vi "STAGE+mono+counter_edit21.vi"() -> ()   [LabVIEW 2017]
panel:
  out "Timeout":bool
  out "PROGRESS":u8(slide) max=10 step=10 scale=0.0..1.0
  in  "?":enum32{"Scan Data", "Scans", "RT Data"}(tab)
  out "XY Graph":cluster{dbl[], dbl[]}(graph)
  out "XY Graph 2":cluster{dbl[], dbl[]}[](graph)
  in  "Collect Data!":bool
  out "Waveform Graph":waveform(dbl)[](graph)
  out "?":i32(knob) scale=0.0..1000000.0
  out "Photon Counts":dbl
  in  "Wavelength":dbl
  in  "Show Real Time Data":bool
  in  "?":enum32{"DELAY", "COUNTER", "MONO", "PLOT"}(tab)
  out "Final time [ps]":dbl
  out "Current time [ps]":dbl
  out "Initial time [ps]":dbl
  in  "Set this as t0":bool
  in  "Axis":i32=1
  in  "Motor ON":bool
  in  "Motor OFF":bool
  out "Current Position [mm]":dbl
  out "Final Position [mm]":dbl
  in  "Data Points":i32=100
  out "Current Point":i32
  in  "Step Size [um]":i32=10
  in  "Target [mm]":dbl format="%.3f"
  in  "Move":bool
  out "Initial position [mm]":dbl
  in  "GPIB address":string="23"
  in  "Count Mode":u16(ring) items=["A,B for Preset T", "A-B for Preset T", "A+B for Preset T", "A for Preset B"]
  in  "Trigger mode":u16(ring) items=["10 MHz"=0, "Input 2"=2, "Input T"=3]
  in  "Channel A Input":u16(ring)=1 items=["10 MHz", "Input 1"]
  in  "Channel B Input":u16(ring)=2 items=["Input 1"=1, "Input 2"=2]
  in  "Number of Measurements\n to take at one point/ Number of Periods":u16=1 min=1 max=2000 step=1
  in  "Time between measurements\n at one point (s)/Dwell Time":dbl=0.002 min=0.002 max=60.0 step=0.001
  in  "gate mode (CW:0)":i16(slide) scale=0.0..2.0 scale format="%.2f"
  out "Counts":i32
  in  "Integrating time \nin 10^-7 sec":dbl=10000000.0
  in  "Discriminator Level (mV)":dbl min=-300.0 max=300.0 step=0.2
  in  "Discriminator Slope":bool
  in  "Channel":i16 min=0 max=2 step=1
  out "Grating #":dbl
  out "Blaze angle":dbl
  out "Grooves/mm":dbl
  out "Mono port":T1(ring)
  out "Time delay":u32=450000 min=1
  in  "Step size":dbl=10.0 min=0.0
  in  "Scan to":i32=4000
  in  "Scan from":i32=2600
  out "Current wavelength":dbl
  in  "?":bool
  in  "Array":dbl[](array[numeric])
  out "Numeric":i32
  out "Numeric 2":i32
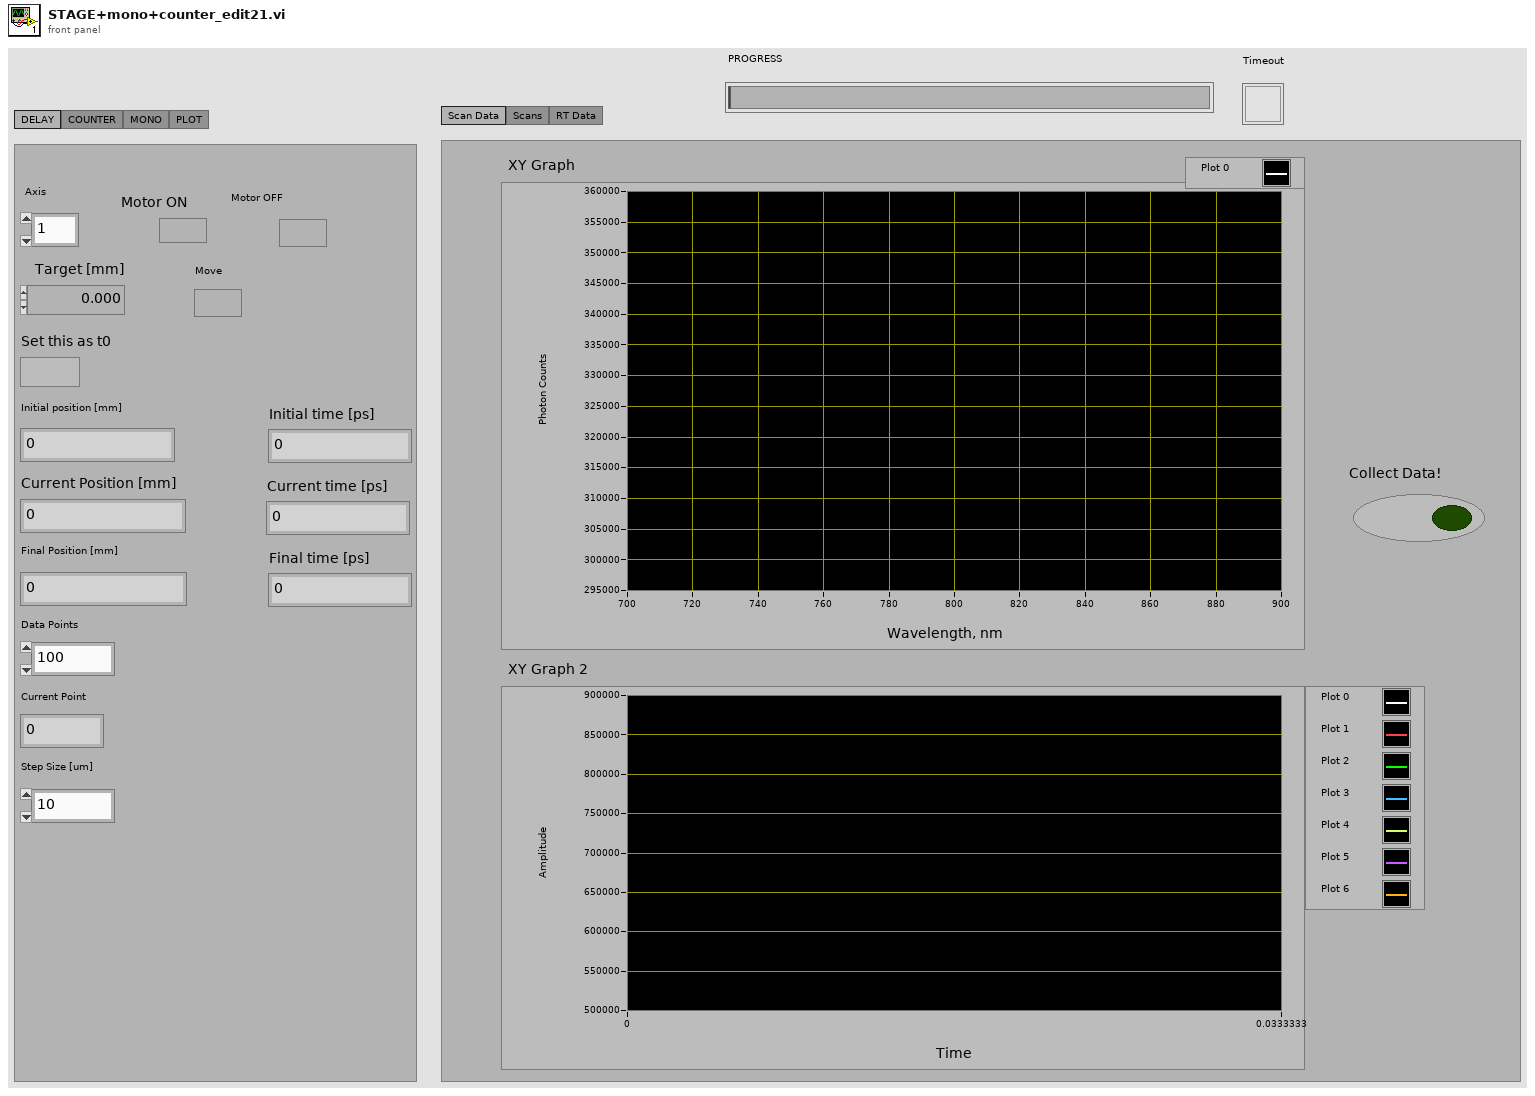
[diagram p1: front panel]
types:
  T1 = enum8{"COM 1", "COM 2", "COM 3", "COM 4", "COM 5", "COM 6", "COM 7", "COM 8", "COM 9"}
  T2 = cluster{"input XON/XOFF":bool, "input HW Handshake":bool, "input alt HW HShk":bool, "output XON/XOFF":bool, "output HW Handshake":bool, "output alt HW HShk":bool, "XOFF byte":u8, "XON byte":u8, "parity error byte":u16}
  T3 = enum16{"no parity", "odd parity", "even parity", "mark parity", "space parity"}
  T4 = typedef "NI_Matrix.lvlib/RealMatrix.ctl" = dbl[][]
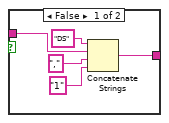
[diagram p3: hidden frame]
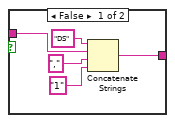
[diagram p5: hidden frame]
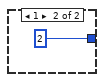
[diagram p9: hidden frame]
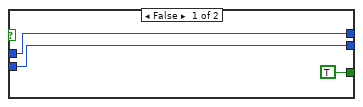
[diagram p10: hidden frame]
diagram:
  (unwired) FALSE
  w28 = u32 19200  # baud rate
  w27 = u16 8  # data bits
  w26 = enum16{"1 bit", "1.5 bits", "2 bits"}."1 bit"  # stop bits
  w30 = T3."no parity"  # parity
  w6 = 4  # 0=COM1 so n=COM(n+1)
  w29 = u16 1024  # buffer size
  n1 = flat-sequence {
    tunnel: [w33] -> w21
    tunnel: [w32] -> w20
    frame #0 {
      n2 = call "CM Com Read ini.vi"() -> ("Mono port"=w32:T1, "time delay1"=w33:u32)  [unwired: 7 in]
    }
  }
  n3 = call "CM Serial Port Setup.vi"("COM port"=w20, "time delay"=w21) -> ("time delay1"=w16:u32, "DK port Out"=w17:T1, "error code"=w19:i32)  [unwired: 7 in]
  n4 = Equal To 0?(x=w19) -> (x = 0?=w18:bool)
  n5 = case shown="True" w18 {
    tunnel: w17 -> [w36 w39]
    tunnel: w16 -> [w35 w38]
    tunnel: [w36 w39] -> w3
    tunnel: [w35 w38] -> w2
    tunnel: [TRUE FALSE] -> w1
    frame False {
    }
    frame True {
      n6 = call "CM Com Write ini.vi"("time delay1"=w39, "Mono port"=w38) -> ()  [unwired: 7 in]
      n7 = local write "Mono port"(w39) -> ()
      n8 = local write "Time delay"(w38) -> ()
    }
  }
  n9 = call <vilib>:"Serial Port Init.vi"("flow control etc."=T2 {"input XON/XOFF"=FALSE, "input HW Handshake"=FALSE, "input alt HW HShk"=FALSE, "output XON/XOFF"=FALSE, "output HW Handshake"=FALSE, "output alt HW HShk"=FALSE, "XOFF byte"=13, "XON byte"=11, "parity error byte"=0}, "parity"=w30, "buffer size"=w29, "stop bits"=w26, "data bits"=w27, "baud rate"=w28, "port number"=w6) -> ("error code"=w25:i32)
  n10 = Concatenate Strings("\r", "\n") -> (w22:string)
  n11 = while {
    tunnel: w2 -> [w42]
    tunnel: w3 -> [w41]
    stop <- TRUE continue-if-true
    n12 = case shown="True" "?" {
      tunnel: w42 -> [_ w45]
      tunnel: w41 -> [_ w44]
      frame False {
      }
      frame True {
        n13 = Two Button Dialog(message="Do you want to change grating?", 1:"No" ("F button name (\"Cancel\")"), 2:"Yes" ("T button name (\"OK\")")) -> (T button?=w46:bool)
        n14 = case shown="True" w46 {
          tunnel: w45 -> [_ w51]
          tunnel: w44 -> [_ w50]
          frame False {
          }
          frame True {
            n15 = Two Button Dialog(message="Disable voltage from PMT", 1:"Do not swich grating" ("F button name (\"Cancel\")"), 2:"Done" ("T button name (\"OK\")")) -> (T button?=w52:bool)
            n16 = case shown="True" w52 {
              tunnel: w51 -> [_ w64]
              tunnel: w50 -> [_ w63]
              frame False {
              }
              frame True {
                n17 = flat-sequence {
                  tunnel: w64 -> [w68]
                  tunnel: [w68] -> w58
                  tunnel: w63 -> [w67]
                  tunnel: [w67] -> w57
                  tunnel: [w65] -> w56
                  tunnel: w58 -> [w73]
                  tunnel: [w73] -> w61
                  tunnel: w57 -> [w74]
                  tunnel: [w74] -> w60
                  tunnel: w56 -> [w72]
                  tunnel: [w72] -> w59
                  tunnel: w61 -> [w78]
                  tunnel: w60 -> [w79]
                  tunnel: [w77] -> w62
                  tunnel: w59 -> [w77]
                  frame #0 {
                    n18 = local read "Grating #"() -> (w66:dbl)
                    n19 = case shown="2, Default" w66 {
                      tunnel: [1 2] -> w65
                      frame 2, Default {
                      }
                      frame 1 {
                      }
                    }
                    n20 = call "Select11x2.vi"("time delay"=w68, "NEW GRT?"=w65, "port number"=w67) -> ()  [unwired: 3 out]
                  }
                  frame #1 {
                    n21 = call "Query11x.vi"("port number"=w74, "QUERY"=u16 2, "time delay"=w73) -> ("STATUS MESSAGE"=w71:u16)  [unwired: 3 out]
                    n22 = local write "Grooves/mm"(w71) -> ()
                  }
                  frame #2 {
                    n23 = Divide(x=w78, y=i16 100 ("device (1)")) -> (x/y=w80:dbl)
                    n24 = call "Query11x.vi"("port number"=w79, "QUERY"=u16 3, "time delay"=w80) -> ("STATUS MESSAGE"=w76:u16)  [unwired: 3 out]
                    n25 = local write "Blaze angle"(w76) -> ()
                  }
                }
                n26 = local write "Grating #"(w62) -> ()
              }
            }
          }
        }
      }
    }
  }
  n27 = while {
    tunnel: w6 -> [w97]
    tunnel: w22 -> [w98]
    tunnel: w25 -> [_]
    tunnel: "Axis" -> [w95]
    stop <- TRUE continue-if-true
    w96 = u32 200  # timeout
    n28 = Format Into String(w95) -> (resulting string=w99:string)  [unwired: 3 in, 1 out]
    n29 = flat-sequence {
      tunnel: w99 -> [w104]
      tunnel: w98 -> [w103]
      tunnel: w97 -> [w105]
      tunnel: w96 -> [w102]
      tunnel: [w104] -> w94
      tunnel: [w103] -> w93
      tunnel: [w105] -> w92
      tunnel: [w102] -> w91
      tunnel: w94 -> [w115]
      tunnel: w93 -> [w114]
      tunnel: w92 -> [w116]
      tunnel: w91 -> [w112]
      tunnel: [w115] -> w90
      tunnel: [w114] -> w89
      tunnel: [w116] -> w88
      tunnel: [w112] -> w87
      tunnel: w90 -> [w125]
      tunnel: w89 -> [w124]
      tunnel: w88 -> [w126]
      tunnel: w87 -> [w122]
      tunnel: [w125] -> w86
      tunnel: [w124] -> w85
      tunnel: [w126] -> w84
      tunnel: [w122] -> w83
      tunnel: w86 -> [w138]
      tunnel: w85 -> [w135]
      tunnel: w84 -> [w137]
      tunnel: w83 -> [w136]
      frame #0 {
        n30 = case shown="True" "Motor ON" {
          tunnel: w105 -> [_ w111]
          tunnel: w104 -> [_ w108]
          tunnel: w103 -> [_ w107]
          frame False {
          }
          frame True {
            n31 = Concatenate Strings(w108, "MO" ("Substring"), w107) -> (w109:string)
            n32 = call <vilib>:"Serial Port Write.vi"("string to write"=w109, "port number"=w111) -> ()  [unwired: 1 out]
          }
        }
      }
      frame #1 {
        n33 = case shown="True" "Motor OFF" {
          tunnel: w116 -> [_ w121]
          tunnel: w115 -> [_ w118]
          tunnel: w114 -> [_ w117]
          frame False {
          }
          frame True {
            n34 = Concatenate Strings(w118, "MF" ("Substring"), w117) -> (w119:string)
            n35 = call <vilib>:"Serial Port Write.vi"("string to write"=w119, "port number"=w121) -> ()  [unwired: 1 out]
          }
        }
      }
      frame #2 {
        n36 = case shown="True" "Move" {
          tunnel: w126 -> [_ w133]
          tunnel: w125 -> [_ w130]
          tunnel: w124 -> [_ w129]
          frame False {
          }
          frame True {
            n37 = Format Into String("Target [mm]") -> (resulting string=w127:string)  [unwired: 3 in, 1 out]
            n38 = Concatenate Strings(w130, "PA" ("Substring"), w127, w129) -> (w131:string)
            n39 = call <vilib>:"Serial Port Write.vi"("string to write"=w131, "port number"=w133) -> ()  [unwired: 1 out]
          }
        }
      }
      frame #3 {
        n40 = case shown="True" "Set this as t0" {
          tunnel: w138 -> [_ w148]
          tunnel: w137 -> [_ w147]
          tunnel: w136 -> [_ w146]
          tunnel: w135 -> [_ w145]
          frame False {
          }
          frame True {
            n41 = flat-sequence {
              tunnel: w148 -> [w152]
              tunnel: w147 -> [w151]
              tunnel: [w151] -> w144
              tunnel: w146 -> [w149]
              tunnel: [w149] -> w143
              tunnel: w145 -> [w150]
              tunnel: w144 -> [w156]
              tunnel: [w156] -> w142
              tunnel: w143 -> [w155]
              tunnel: [w155] -> w141
              tunnel: [w157] -> w140
              tunnel: w142 -> [w162]
              tunnel: w141 -> [w160]
              tunnel: w140 -> [w159]
              tunnel: [w158] -> w139
              tunnel: w139 -> [w184]
              frame #0 {
                # "send position query"
                n42 = Concatenate Strings(w152, "TP" ("Substring"), w150) -> (w153:string)
                n43 = call <vilib>:"Serial Port Write.vi"("string to write"=w153, "port number"=w151) -> ()  [unwired: 1 out]
              }
              frame #1 {
                # "record current time"
                n44 = Tick Count (ms)() -> (millisecond timer value=w157:u32)
              }
              frame #2 {
                # "read characters in serial port"
                n45 = while {
                  shift-left: w159 -> [w163]
                  shift-right: [w164] -> _
                  tunnel: w160 -> [w167]
                  shift-left: "" -> [w170]
                  shift-right: [w169] -> w158
                  tunnel: w162 -> [w171]
                  stop <- w166 continue-if-true
                  n46 = call <vilib>:"Bytes At Serial Port.vi"("port number"=w171) -> ("byte count"=w172:u32)  [unwired: 1 out]
                  n47 = Tick Count (ms)() -> (millisecond timer value=w165:u32)
                  n48 = Subtract(x=w165, y=w163) -> (x-y=w168:u32)
                  n49 = Greater Than 0?(x=w172) -> (x > 0?=w173:bool)
                  n50 = Less?(x=w168, y=w167) -> (x < y?=w166:bool)
                  n51 = case shown="True" w173 {
                    tunnel: w172 -> [_ w181]
                    tunnel: w171 -> [_ w180]
                    tunnel: w170 -> [w175 w178]
                    tunnel: [w175 w177] -> w169
                    tunnel: [w174 w176] -> w164
                    tunnel: w165 -> [_ w176]
                    tunnel: w163 -> [w174 _]
                    frame False {
                    }
                    frame True {
                      n52 = call <vilib>:"Serial Port Read.vi"("requested byte count"=w181, "port number"=w180) -> ("string read"=w179:string)  [unwired: 1 out]
                      n53 = Concatenate Strings(w178, w179) -> (w177:string)
                    }
                  }
                }
              }
              frame #3 {
                n54 = Scan From String(input string=w184) -> (output 1=w182:dbl)  [unwired: 4 in, 3 out]
                n55 = Subtract(x=w182, y=w182) -> (x-y=→"Initial position [mm]":dbl)
              }
            }
          }
        }
      }
    }
    n56 = Wait Until Next ms Multiple(millisecond multiple=u32 50) -> ()  [unwired: 1 out]
  }
  n57 = while {
    tunnel: "GPIB address" -> [w188]
    tunnel: w3 -> [w187]
    tunnel: w2 -> [w186]
    tunnel: w1 -> [w185]
    stop <- TRUE continue-if-true
    n58 = case shown="True" "Show Real Time Data" {
      tunnel: w188 -> [_ w195]
      tunnel: w187 -> [_ w194]
      tunnel: w186 -> [_ w193]
      tunnel: w185 -> [_ w192]
      frame False {
      }
      frame True {
        n59 = flat-sequence {
          tunnel: w195 -> [w224]
          tunnel: "Wavelength" -> [w225]
          tunnel: [w225] -> w206
          tunnel: [w214] -> w205
          tunnel: [w213] -> w204
          tunnel: [w224] -> w203
          tunnel: w193 -> [w217]
          tunnel: w194 -> [w216]
          tunnel: w192 -> [w215]
          tunnel: [w264] -> w202
          tunnel: [w263] -> w201
          tunnel: [w261] -> w200
          tunnel: w206 -> [w259]
          tunnel: w205 -> [w264]
          tunnel: w204 -> [w263]
          tunnel: w203 -> [w261]
          tunnel: w202 -> [w271]
          tunnel: w201 -> [w270]
          tunnel: w200 -> [w265]
          tunnel: [w265] -> w199
          tunnel: w199 -> [w276]
          tunnel: [w276] -> w198
          tunnel: w198 -> [w326]
          tunnel: [w326] -> w197
          tunnel: w197 -> [w327]
          tunnel: [w327] -> w196
          tunnel: w196 -> [w337]
          frame #0 {
            n60 = flat-sequence {
              tunnel: w217 -> [w231]
              tunnel: [w231] -> w223
              tunnel: w216 -> [w233]
              tunnel: [w233] -> w222
              tunnel: w215 -> [w229]
              tunnel: [w229] -> w221
              tunnel: w223 -> [w237]
              tunnel: [w237] -> w212
              tunnel: w222 -> [w238]
              tunnel: [w238] -> w210
              tunnel: w221 -> [w235]
              tunnel: [w235] -> w208
              tunnel: w212 -> [w242]
              tunnel: [w242] -> w211
              tunnel: w210 -> [w241]
              tunnel: [w241] -> w209
              tunnel: w208 -> [w240]
              tunnel: [w240] -> w207
              tunnel: w211 -> [w249]
              tunnel: [w249] -> w220
              tunnel: w209 -> [w246]
              tunnel: [w246] -> w219
              tunnel: w207 -> [w244]
              tunnel: [w244] -> w218
              tunnel: w220 -> [w252]
              tunnel: w219 -> [w253]
              tunnel: w218 -> [_]
              tunnel: [w253] -> w214
              tunnel: [w252] -> w213
              frame #0 {
                n61 = call "Query11x.vi"("port number"=w233, "QUERY"=u16 0, "time delay"=w231) -> ("timeout"=w230:bool, "STATUS MESSAGE"=w228:u16)  [unwired: 2 out]
                n62 = local write "Timeout"(w230) -> ()
                n63 = Divide(x=w228, y=10 ("Numeric")) -> (x/y=w226:dbl)
                n64 = local write "Current wavelength"(w226) -> ()
              }
              frame #1 {
                n65 = call "Query11x.vi"("port number"=w238, "QUERY"=u16 2, "time delay"=w237) -> ("timeout"=w236:bool, "STATUS MESSAGE"=w234:u16)  [unwired: 2 out]
                n66 = local write "Timeout"(w236) -> ()
                n67 = local write "Grooves/mm"(w234) -> ()
              }
              frame #2 {
              }
              frame #3 {
                n68 = Divide(x=w249, y=i16 100 ("device (1)")) -> (x/y=w247:dbl)
                n69 = call "Query11x.vi"("port number"=w246, "QUERY"=u16 3, "time delay"=w247) -> ("timeout"=w245:bool, "STATUS MESSAGE"=w243:u16)  [unwired: 2 out]
                n70 = local write "Timeout"(w245) -> ()
                n71 = local write "Blaze angle"(w243) -> ()
              }
              frame #4 {
                n72 = Divide(x=w252, y=i16 100 ("device (1)")) -> (x/y=w255:dbl)
                n73 = call "Query11x.vi"("port number"=w253, "QUERY"=u16 4, "time delay"=w255) -> ("timeout"=w254:bool, "STATUS MESSAGE"=w251:u16)  [unwired: 2 out]
                n74 = local write "Timeout"(w254) -> ()
                n75 = local write "Grating #"(w251) -> ()
              }
            }
          }
          frame #1 {
            n76 = Multiply(x=w259, y=10) -> (x*y=w258:dbl)
            n77 = call "Goto11x.vi"("time delay"=w263, "WAVELENGTH"=w258, "port number"=w264) -> ("timeout"=w262:bool)  [unwired: 2 out]
            n78 = local write "Timeout"(w262) -> ()
          }
          frame #2 {
            # "set counter time in 10^-7 seconds in CW"
            n79 = call "Query11x.vi"("port number"=w271, "QUERY"=0, "time delay"=w270) -> ("timeout"=w269:bool, "STATUS MESSAGE"=w268:u16)  [unwired: 2 out]
            n80 = local write "Timeout"(w269) -> ()
            n81 = Divide(x=w268, y=10) -> (x/y=w267:dbl)
            n82 = local write "Current wavelength"(w267) -> ()
          }
          frame #3 {
            # "Configures discriminator."
            n83 = flat-sequence {
              tunnel: w276 -> [w283]
              tunnel: [w283] -> w282
              tunnel: [w290] -> w281
              tunnel: [w288] -> w280
              tunnel: w275 -> [w289]
              tunnel: w282 -> [w288]
              tunnel: w277 -> [w287]
              tunnel: w281 -> [w309]
              tunnel: [w310] -> w279
              tunnel: w280 -> [w308]
              tunnel: [w308] -> w278
              tunnel: w277 -> [w306]
              tunnel: w279 -> [w322]
              tunnel: w278 -> [w321]
              tunnel: w273 -> [w316]
              tunnel: w277 -> [w315]
              frame #0 {
                # "Flush I/O buffers."
                n84 = for {
                  N: 5 -> [_]
                  tunnel: w283 -> [w285]
                  n85 = GPIB Write(0:w285, 1:"\r") -> ()  [unwired: 3 in, 2 out]
                }
              }
              frame #1 {
                # "Set discriminator slope."
                n86 = case shown="True" w289 {
                  tunnel: [w296 w301] -> w291
                  tunnel: w287 -> [w295 w300]
                  frame False {
                    n87 = Concatenate Strings("DS", w295, ",", "1") -> (w296:string)
                  }
                  frame True {
                    n88 = Concatenate Strings("DS", w300, ",", "0") -> (w301:string)
                  }
                }
                n89 = GPIB Write(0:w288, 1:w291, 2:5) -> (6:w290:errorcluster)  [unwired: 2 in, 1 out]
              }
              frame #2 {
                # "Set discriminator mode to fixed."
                n90 = Concatenate Strings("DM", w306, ",", "0") -> (w305:string)
                n91 = GPIB Write(0:w308, 1:w305, 2:5, 3:w309) -> (6:w310:errorcluster)  [unwired: 1 in, 1 out]
              }
              frame #3 {
                # "Set discriminator level.\nMust be between +300 and -300 mV."
                n92 = Divide(x=w316, y=1000.0) -> (x/y=w324:dbl)
                n93 = Number To Fractional String(number=w324, precision (6)=i16 4) -> (F-format string=w313:string)  [unwired: 2 in]
                n94 = Concatenate Strings("DL", w315, ",", w313) -> (w320:string)
                n95 = GPIB Write(0:w321, 1:w320, 2:5, 3:w322) -> (6:w317:errorcluster)  [unwired: 1 in, 1 out]
                n96 = call <vilib>:"General Error Handler.vi"("type of dialog (OK msg:1)"=1, "error in (no error)"=w317) -> ()  [unwired: 9 in, 5 out]
              }
            }
            n97 = local read "Discriminator Slope"() -> (w275:bool)
            n98 = local read "Channel"() -> (w274:i16)
            n99 = Number To Decimal String(number=w274) -> (decimal integer string=w277:string)  [unwired: 1 in]
            n100 = local read "Discriminator Level (mV)"() -> (w273:dbl)
          }
          frame #4 {
            n101 = call "Start.vi"("GPIB Address"=w326) -> ()  [unwired: 9 in]
          }
          frame #5 {
            # "Wait for Scan to Finish"
            n102 = for {
              N: 1 -> [_]
              tunnel: w327 -> [w329]
              n103 = while {
                tunnel: w329 -> [w330]
                stop <- w332 stop-if-true
                n104 = call "ScanDone.vi"("Wait (ms)"=1000, "GPIB Address"=w330) -> ("Scan Finished?"=w332:bool)
              }
            }
          }
          frame #6 {
            n105 = call "Read Data.vi"("Channel Number"=0, "GPIB Address"=w337, "Number of Datapoints"=1) -> ("Data"=w338:i32[])
            n106 = property class="Knob (strict)"("Scale.Increment"=1000, "Scale.Maximum"=1000000, "Scale.Minimum"=0) -> ()  [unwired: 2 in, 2 out]
            n107 = Index Array(array=w338, index=0) -> (element=→"Photon Counts" →"?":i32)
          }
        }
      }
    }
  }
  n108 = while {
    tunnel: "Axis" -> [w350]
    tunnel: w6 -> [w349]
    tunnel: "GPIB address" -> [w348]
    tunnel: "Integrating time \nin 10^-7 sec" -> [w347]
    tunnel: w2 -> [w346]
    tunnel: w3 -> [w345]
    tunnel: w1 -> [w344]
    stop <- TRUE continue-if-true
    n109 = case shown="True" "Collect Data!" {
      selector: "Collect Data!" -> [_ w351]
      tunnel: w350 -> [_ w359]
      tunnel: w349 -> [_ w358]
      tunnel: w348 -> [_ w357]
      tunnel: w348 -> [_ w355]
      tunnel: w347 -> [_ w354]
      tunnel: w346 -> [_ w353]
      tunnel: w345 -> [_ w356]
      tunnel: w344 -> [_ w352]
      frame False {
      }
      frame True {
        n110 = flat-sequence {
          tunnel: w359 -> [w379]
          tunnel: w358 -> [w377]
          tunnel: w357 -> [w376]
          tunnel: w356 -> [w375]
          tunnel: w355 -> [w374]
          tunnel: w354 -> [w371]
          tunnel: w353 -> [w364]
          tunnel: w352 -> [w363]
          tunnel: w351 -> [_]
          frame #0 {
            w384 = 1000000000000.0
            w389 = 1000
            w390 = 300000000
            w396 = 1
            w407 = "\r\n"
            n111 = Multiply(x="Step Size [um]", y="Data Points") -> (x*y=w393:i32)
            n112 = Divide(x="Step Size [um]", y=1000.0) -> (x/y=w427:dbl)
            n113 = local read "Initial position [mm]"() -> (w381:dbl)
            n114 = Multiply(x="Scan to", y=w396) -> (x*y=w370:i32)
            n115 = Increment(x="Data Points") -> (x+1=w438:i32)
            n116 = Multiply(x="Scan from", y=w396) -> (x*y=w369:i32)
            n117 = Divide(x=w393, y=1000) -> (x/y=w392:dbl)
            n118 = To Time Stamp(1:w369) -> (0:w399:timestamp)
            n119 = Multiply(x=w370, y=1) -> (x*y=w433:i32)
            n120 = Multiply(x=1, y=w369) -> (x*y=w373:i32)
            n121 = Divide(x=w427, y=1000.0) -> (x/y=w428:dbl)
            n122 = for {
              N: w438 -> [_]
              tunnel: w427 -> [w745]
              tunnel: w381 -> [w743]
              tunnel: [w736] -> w437 mode=indexing
              i -> [w744]
              # "distances"
              n123 = Multiply(x=w745, y=w744) -> (x*y=w742:dbl)
              n124 = Add(x=w743, y=w742) -> (x+y=w741:dbl)
              n125 = Divide(x=w741, y=1000) -> (x/y=w735:dbl)
              n126 = Divide(x=w735, y=300000000) -> (x/y=w738:dbl)
              n127 = Multiply(x=w738, y=1000000000000.0) -> (x*y=w736:dbl)
            }
            n128 = Divide(x=w381, y=w389) -> (x/y=w387:dbl)
            n129 = Subtract(x=w433, y=w373) -> (x-y=w444:i32)
            n130 = Add(x=w381, y=w392) -> (x+y=w383:dbl)
            "Final Position [mm]" <- w383
            n131 = property on="Waveform Graph" class="WFGraph (strict)"("XScale.Increment"="Step size", "XScale.Maximum"=w370, "XScale.Minimum"=w369) -> ()  [unwired: 2 in, 2 out]
            n132 = Divide(x=w383, y=w389) -> (x/y=w388:dbl)
            n133 = Divide(x=w387, y=w390) -> (x/y=w386:dbl)
            n134 = Divide(x=w428, y=300000000) -> (x/y=w430:dbl)
            n135 = Divide(x=w444, y="Step size") -> (x/y=w443:dbl)
            n136 = Bundle By Name("Y"=dbl[] [], "t0"=w399, "dt"="Step size") -> (w398:waveform(dbl))  [unwired: 1 in]
            n137 = Divide(x=w388, y=w390) -> (x/y=w385:dbl)
            n138 = Multiply(x=w430, y=1000000000000.0) -> (x*y=w367:dbl)
            n139 = Multiply(x=w386, y=w384) -> (x*y=w366:dbl)
            "Initial time [ps]" <- w366
            n140 = Build Array(w398) -> (w362:waveform(dbl)[])
            n141 = Round Toward -Infinity(1:w443) -> (0:w372:dbl)
            n142 = Concatenate Strings("\r", "\n") -> (w378:string)
            n143 = Multiply(x=w385, y=w384) -> (x*y=w397:dbl)
            "Final time [ps]" <- w397
            n144 = Increment(x=w372) -> (x+1=w426:dbl)
            n145 = for {
              N: w426 -> [_]
              tunnel: "Step size" -> [w750]
              tunnel: w373 -> [w748]
              tunnel: [w746] -> w425 mode=indexing
              i -> [w749]
              # "wavelengths"
              n146 = Multiply(x=w750, y=w749) -> (x*y=w747:dbl)
              n147 = Add(x=w748, y=w747) -> (x+y=w746:dbl)
            }
            n148 = property on="XY Graph 2" class="XYGraph (strict)"("XScale.Increment"=w367, "XScale.Maximum"=w397, "XScale.Minimum"=w366) -> ()  [unwired: 2 in, 2 out]
            n149 = for {
              N: "Data Points" -> [w461]
              tunnel: w381 -> [w506]
              tunnel: "Step Size [um]" -> [w502]
              tunnel: w379 -> [w499]
              tunnel: w378 -> [w496]
              tunnel: w377 -> [w497]
              tunnel: w376 -> [w495]
              tunnel: w375 -> [w493]
              tunnel: w374 -> [w494]
              tunnel: [w471] -> w360 mode=indexing
              tunnel: w373 -> [w451]
              tunnel: "Step size" -> [w488]
              tunnel: w372 -> [w487]
              tunnel: w371 -> [w486]
              tunnel: w370 -> [w485]
              tunnel: w369 -> [w484]
              tunnel: "Step size" -> [w477]
              tunnel: w367 -> [w463]
              tunnel: w366 -> [w482]
              shift-right: [w462] -> _
              shift-left: dbl[] [] -> [w457]
              tunnel: w364 -> [w476]
              tunnel: w375 -> [w475]
              tunnel: w363 -> [w474]
              shift-right: [w468] -> _
              shift-left: w362 -> [w469]
              shift-right: [w455] -> _
              shift-left: dbl[][] [] -> [w454]
              i -> [w460]
              w473 = dbl[] []
              n150 = property on="PROGRESS" class="Slide (strict)"("Scale.Increment"=1, "Scale.Maximum"=w461, "Scale.Minimum"=0) -> ()  [unwired: 2 in, 2 out]
              n151 = stacked-sequence {
                tunnel: w493 -> [w718]
                tunnel: w494 -> [_]
                frame #0 {
                  n152 = call <vilib>:"Close Serial Driver.vi"("port number"=w718) -> ()  [unwired: 1 out]
                  n153 = GPIB Misc(0:"loc 23" ("command string")) -> ()  [unwired: 1 in, 3 out]
                }
              }
              n154 = flat-sequence {
                tunnel: w495 -> [w528]
                tunnel: w451 -> [w527]
                tunnel: w488 -> [w526]
                tunnel: w487 -> [w525]
                tunnel: w485 -> [w524]
                tunnel: w484 -> [w523]
                tunnel: w473 -> [w522]
                tunnel: w473 -> [w521]
                tunnel: w477 -> [w520]
                tunnel: w476 -> [w519]
                tunnel: w475 -> [w518]
                tunnel: w474 -> [w517]
                tunnel: [w515] -> w472
                tunnel: [w516] -> _
                tunnel: [w515] -> w470
                tunnel: [w698] -> w471
                tunnel: w472 -> [w698]
                tunnel: [w697] -> w456
                tunnel: [w696] -> w453
                frame #0 {
                  # "step size"
                  n155 = while {
                    tunnel: w528 -> [w538]
                    tunnel: w527 -> [w562]
                    tunnel: w526 -> [w531]
                    tunnel: w525 -> [w561]
                    tunnel: w524 -> [w534]
                    tunnel: w523 -> [w533]
                    tunnel: w520 -> [w535]
                    shift-right: [w557] -> w515
                    shift-left: w521 -> [w556]
                    shift-right: [w552] -> w516
                    shift-left: w522 -> [w559]
                    tunnel: w519 -> [w542]
                    tunnel: w518 -> [w541]
                    tunnel: w517 -> [w540]
                    i -> [w560]
                    stop <- w529 stop-if-true
                    n156 = property on="XY Graph" class="XYGraph (strict)"("XScale.Increment"=w535, "XScale.Maximum"=w534, "XScale.Minimum"=w533) -> ()  [unwired: 2 in, 2 out]
                    n157 = Multiply(x=1, y=w531) -> (x*y=w530:dbl)
                    n158 = Multiply(x=w560, y=w530) -> (x*y=w563:dbl)
                    n159 = Greater Or Equal?(x=w560, y=w561) -> (x >= y?=w529:bool)
                    n160 = Add(x=w563, y=w562) -> (x+y=w539:dbl)
                    n161 = Build Array (concatenate)(w559, w539) -> (w558:dbl[])
                    n162 = flat-sequence {
                      tunnel: w538 -> [w581]
                      tunnel: w539 -> [w582]
                      tunnel: [w582] -> w546
                      tunnel: [w571] -> w545
                      tunnel: [w570] -> w544
                      tunnel: [w581] -> w543
                      tunnel: w542 -> [w574]
                      tunnel: w541 -> [w573]
                      tunnel: w540 -> [w572]
                      tunnel: [w621] -> w551
                      tunnel: [w620] -> w550
                      tunnel: [w618] -> w549
                      tunnel: w546 -> [w616]
                      tunnel: w545 -> [w621]
                      tunnel: w544 -> [w620]
                      tunnel: w543 -> [w618]
                      tunnel: w551 -> [w628]
                      tunnel: w550 -> [w627]
                      tunnel: w549 -> [w622]
                      tunnel: [w622] -> w537
                      tunnel: w537 -> [w630]
                      tunnel: [w630] -> w536
                      tunnel: w536 -> [w683]
                      tunnel: [w683] -> w548
                      tunnel: w548 -> [w684]
                      tunnel: [w684] -> w547
                      tunnel: [w690] -> w554
                      tunnel: w547 -> [w691]
                      frame #0 {
                        n163 = flat-sequence {
                          tunnel: w574 -> [w588]
                          tunnel: [w588] -> w580
                          tunnel: w573 -> [w590]
                          tunnel: [w590] -> w579
                          tunnel: w572 -> [w586]
                          tunnel: [w586] -> w578
                          tunnel: w580 -> [w594]
                          tunnel: [w594] -> w569
                          tunnel: w579 -> [w595]
                          tunnel: [w595] -> w567
                          tunnel: w578 -> [w592]
                          tunnel: [w592] -> w565
                          tunnel: w569 -> [w599]
                          tunnel: [w599] -> w568
                          tunnel: w567 -> [w598]
                          tunnel: [w598] -> w566
                          tunnel: w565 -> [w597]
                          tunnel: [w597] -> w564
                          tunnel: w568 -> [w606]
                          tunnel: [w606] -> w577
                          tunnel: w566 -> [w603]
                          tunnel: [w603] -> w576
                          tunnel: w564 -> [w601]
                          tunnel: [w601] -> w575
                          tunnel: w577 -> [w608]
                          tunnel: w576 -> [w609]
                          tunnel: w575 -> [_]
                          tunnel: [w609] -> w571
                          tunnel: [w608] -> w570
                          frame #0 {
                            n164 = call "Query11x.vi"("port number"=w590, "QUERY"=u16 0, "time delay"=w588) -> ("timeout"=w587:bool, "STATUS MESSAGE"=w585:u16)  [unwired: 2 out]
                            n165 = local write "Timeout"(w587) -> ()
                            n166 = Divide(x=w585, y=10 ("Numeric")) -> (x/y=→"Current wavelength":dbl)
                          }
                          frame #1 {
                            n167 = call "Query11x.vi"("port number"=w595, "QUERY"=u16 2, "time delay"=w594) -> ("timeout"=w593:bool, "STATUS MESSAGE"=→"Grooves/mm":u16)  [unwired: 2 out]
                            n168 = local write "Timeout"(w593) -> ()
                          }
                          frame #2 {
                          }
                          frame #3 {
                            n169 = Divide(x=w606, y=i16 100 ("device (1)")) -> (x/y=w604:dbl)
                            n170 = call "Query11x.vi"("port number"=w603, "QUERY"=u16 3, "time delay"=w604) -> ("timeout"=w602:bool, "STATUS MESSAGE"=→"Blaze angle":u16)  [unwired: 2 out]
                            n171 = local write "Timeout"(w602) -> ()
                          }
                          frame #4 {
                            n172 = Divide(x=w608, y=i16 100 ("device (1)")) -> (x/y=w612:dbl)
                            n173 = call "Query11x.vi"("port number"=w609, "QUERY"=u16 4, "time delay"=w612) -> ("timeout"=w611:bool, "STATUS MESSAGE"=→"Grating #":u16)  [unwired: 2 out]
                            n174 = local write "Timeout"(w611) -> ()
                          }
                        }
                      }
                      frame #1 {
                        n175 = Multiply(x=w616, y=10) -> (x*y=w615:dbl)
                        n176 = call "Goto11x.vi"("time delay"=w620, "WAVELENGTH"=w615, "port number"=w621) -> ("timeout"=w619:bool)  [unwired: 2 out]
                        n177 = local write "Timeout"(w619) -> ()
                      }
                      frame #2 {
                        # "set counter time in 10^-7 seconds in CW"
                        n178 = call "Query11x.vi"("port number"=w628, "QUERY"=0, "time delay"=w627) -> ("timeout"=w626:bool, "STATUS MESSAGE"=w625:u16)  [unwired: 2 out]
                        n179 = local write "Timeout"(w626) -> ()
                        n180 = Divide(x=w625, y=10) -> (x/y=w624:dbl)
                        n181 = local write "Current wavelength"(w624) -> ()
                      }
                      frame #3 {
                        # "Configures discriminator."
                        n182 = flat-sequence {
                          tunnel: w630 -> [w640]
                          tunnel: [w640] -> w639
                          tunnel: [w647] -> w638
                          tunnel: [w645] -> w637
                          tunnel: "Discriminator Slope" -> [w646]
                          tunnel: w639 -> [w645]
                          tunnel: w631 -> [w644]
                          tunnel: w638 -> [w666]
                          tunnel: [w667] -> w636
                          tunnel: w637 -> [w665]
                          tunnel: [w665] -> w635
                          tunnel: w631 -> [w663]
                          tunnel: w636 -> [w679]
                          tunnel: w635 -> [w678]
                          tunnel: "Discriminator Level (mV)" -> [w673]
                          tunnel: w631 -> [w672]
                          frame #0 {
                            # "Flush I/O buffers."
                            n183 = for {
                              N: 5 -> [_]
                              tunnel: w640 -> [w642]
                              n184 = GPIB Write(0:w642, 1:"\r") -> ()  [unwired: 3 in, 2 out]
                            }
                          }
                          frame #1 {
                            # "Set discriminator slope."
                            n185 = case shown="True" w646 {
                              tunnel: [w653 w658] -> w648
                              tunnel: w644 -> [w652 w657]
                              frame False {
                                n186 = Concatenate Strings("DS", w652, ",", "1") -> (w653:string)
                              }
                              frame True {
                                n187 = Concatenate Strings("DS", w657, ",", "0") -> (w658:string)
                              }
                            }
                            n188 = GPIB Write(0:w645, 1:w648, 2:5) -> (6:w647:errorcluster)  [unwired: 2 in, 1 out]
                          }
                          frame #2 {
                            # "Set discriminator mode to fixed."
                            n189 = Concatenate Strings("DM", w663, ",", "0") -> (w662:string)
                            n190 = GPIB Write(0:w665, 1:w662, 2:5, 3:w666) -> (6:w667:errorcluster)  [unwired: 1 in, 1 out]
                          }
                          frame #3 {
                            # "Set discriminator level.\nMust be between +300 and -300 mV."
                            n191 = Divide(x=w673, y=1000.0) -> (x/y=w681:dbl)
                            n192 = Number To Fractional String(number=w681, precision (6)=i16 4) -> (F-format string=w670:string)  [unwired: 2 in]
                            n193 = Concatenate Strings("DL", w672, ",", w670) -> (w677:string)
                            n194 = GPIB Write(0:w678, 1:w677, 2:5, 3:w679) -> (6:w674:errorcluster)  [unwired: 1 in, 1 out]
                            n195 = call <vilib>:"General Error Handler.vi"("type of dialog (OK msg:1)"=1, "error in (no error)"=w674) -> ()  [unwired: 9 in, 5 out]
                          }
                        }
                        n196 = Number To Decimal String(number="Channel") -> (decimal integer string=w631:string)  [unwired: 1 in]
                      }
                      frame #4 {
                        n197 = call "Start.vi"("GPIB Address"=w683) -> ()  [unwired: 9 in]
                      }
                      frame #5 {
                        # "Wait for Scan to Finish"
                        n198 = for {
                          N: 1 -> [_]
                          tunnel: w684 -> [w686]
                          n199 = while {
                            tunnel: w686 -> [w687]
                            stop <- w689 stop-if-true
                            n200 = call "ScanDone.vi"("Wait (ms)"=1000, "GPIB Address"=w687) -> ("Scan Finished?"=w689:bool)
                          }
                        }
                      }
                      frame #6 {
                        n201 = call "Read Data.vi"("Channel Number"=0, "GPIB Address"=w691, "Number of Datapoints"=1) -> ("Data"=w692:i32[])
                        n202 = Index Array(array=w692, index=0) -> (element=w690:i32)
                        "Counts" <- w690
                      }
                    }
                    n203 = Build Array (concatenate)(w556, w554) -> (w555:dbl[])
                    n204 = Bundle(w558, w555) -> (w553:cluster{dbl[], dbl[]})  [unwired: 1 in]
                    "XY Graph" <- w553
                    n205 = Unbundle(w553) -> (w552:dbl[], w557:dbl[])
                  }
                }
                frame #1 {
                  n206 = Array Size(array="Array") -> (size(s)=w696:i32)
                  n207 = flat-sequence {
                    tunnel: w698 -> [w704]
                    tunnel: "Array" -> [w703]
                    tunnel: w696 -> [w702]
                    tunnel: [w700] -> w697
                    frame #0 {
                      n208 = for {
                        N: w702 -> [w709]
                        tunnel: w703 -> [w716]
                        tunnel: w704 -> [w711]
                        shift-right: [w705] -> w700
                        shift-left: dbl[] [] -> [w706]
                        i -> [w708]
                        n209 = local read "Scan from"() -> (w714:i32)
                        n210 = Index Array(array=w716, index=w708) -> (element=w715:dbl)
                        n211 = local read "Step size"() -> (w712:dbl)
                        n212 = Subtract(x=w715, y=w714) -> (x-y=w713:dbl)
                        n213 = Divide(x=w713, y=w712) -> (x/y=w710:dbl)
                        n214 = Index Array(array=w711, index=w710) -> (element=w707:dbl)
                        n215 = Insert Into Array(array=w706, index=w708, new element=w707) -> (w705:dbl[])
                        "Numeric" <- w709
                      }
                    }
                  }
                }
              }
              n216 = Multiply(x=w463, y=w460) -> (x*y=w483:dbl)
              n217 = Number To Decimal String(number=w486) -> (decimal integer string=w491:string)  [unwired: 1 in]
              n218 = Add(x=1, y=w460) -> (x+y=→"PROGRESS":i32)
              n219 = Divide(x=w502, y=1000) -> (x/y=w501:dbl)
              n220 = Add(x=w482, y=w483) -> (x+y=w458:dbl)
              n221 = Concatenate Strings("CP 2,", w491) -> (w489:string)
              n222 = Multiply(x=w501, y=w460) -> (x*y=w505:dbl)
              n223 = Build Array (concatenate)(w457, w458) -> (w459:dbl[])
              n224 = Add(x=w506, y=w505) -> (x+y=w504:dbl)
              n225 = Format Into String(w499) -> (resulting string=w498:string)  [unwired: 3 in, 1 out]
              n226 = GPIB Write(0:w495, 1:w489, 2:i16 5 ("mode (0)")) -> ()  [unwired: 2 in, 2 out]
              n227 = flat-sequence {
                tunnel: w504 -> [w721]
                tunnel: [w721] -> w500
                tunnel: w496 -> [w723]
                tunnel: w498 -> [w722]
                tunnel: w497 -> [w719]
                tunnel: w500 -> [w732]
                frame #0 {
                  n228 = Format Into String(w721) -> (resulting string=w720:string)  [unwired: 3 in, 1 out]
                  n229 = Wait (ms)(milliseconds to wait=u32 100) -> ()  [unwired: 1 out]
                  n230 = Concatenate Strings(w722, "PA" ("Substring"), w720, w723) -> (w725:string)
                  n231 = call <vilib>:"Serial Port Write.vi"("string to write"=w725, "port number"=w719) -> ()  [unwired: 1 out]
                }
                frame #1 {
                  n232 = Divide(x=w732, y=1000) -> (x/y=w730:dbl)
                  n233 = Wait (ms)(milliseconds to wait=u32 1000) -> ()  [unwired: 1 out]
                  n234 = Divide(x=w730, y=300000000) -> (x/y=w729:dbl)
                  n235 = Multiply(x=w729, y=1000000000000.0) -> (x*y=→"Current time [ps]":dbl)
                  "Current Position [mm]" <- w732
                }
              }
              n236 = local read "Scan from"() -> (w466:i32)
              n237 = local read "Step size"() -> (w464:dbl)
              n238 = To Time Stamp(1:w466) -> (0:w465:timestamp)
              n239 = Bundle By Name("Y"=w470, "t0"=w465, "dt"=w464) -> (w467:waveform(dbl))  [unwired: 1 in]
              n240 = Build Array (concatenate)(w469, w467) -> (w468:waveform(dbl)[])
              "Waveform Graph" <- w468
              n241 = for {
                N: w453 -> [_]
                tunnel: [w514] -> w462
                tunnel: w459 -> [w513]
                tunnel: w456 -> [w511]
                tunnel: [w510] -> w455
                tunnel: w454 -> [w512]
                tunnel: [w507] -> w452 mode=indexing
                i -> [w509]
                n242 = Build Array (concatenate)(w512, w511) -> (w510:dbl[][])
                n243 = Index Array(array=w511, index=w509) -> ()  [unwired: 1 out]
                n244 = Index Array(array=w510, index (col)=w509) -> (element=w508:dbl[])  [unwired: 1 in]
                n245 = Bundle(w513, w508) -> (w507:cluster{dbl[], dbl[]})  [unwired: 1 in]
                n246 = Unbundle(w507) -> (w514:dbl[])  [unwired: 1 out]
              }
              "XY Graph 2" <- w452
              "Current Point" <- w460
              "Numeric 2" <- w461
            }
            n247 = Build Array (concatenate)(0, w437) -> (w401:dbl[])
            n248 = local read "Integrating time \nin 10^-7 sec"() -> (w405:dbl)
            n249 = Build Array(w425) -> (w442:dbl[][])
            n250 = Transpose Matrix(1:w442) -> (0:w441:dbl[][])
            n251 = Transpose Matrix(1:w360) -> (0:w440:dbl[][])
            n252 = Build Array (concatenate)(w441, w440) -> (w402:T4)
            n253 = Insert Into Array(array=w402, index (row)=0, new element=w401) -> (w434:T4)  [unwired: 1 in]
            n254 = local read "Blaze angle"() -> (w424:dbl)
            n255 = local read "Grating #"() -> (w423:dbl)
            n256 = Multiply(x=w405, y=1e-07) -> (x*y=w404:dbl)
            n257 = Get Date/Time In Seconds() -> (seconds since 1Jan1904=w417:timestamp)
            n258 = Array To Spreadsheet String(delimiter (Tab)=",", array=w434, 3:"%f" ("format string")) -> (spreadsheet string=w406:string)
            n259 = Format Date/Time String(time format string (%c)="%Y-%b-%d %H:%M:%S", seconds (now)=w417) -> (date/time string=w418:string)  [unwired: 1 in]
            n260 = Number To Decimal String(number=w404) -> (decimal integer string=w419:string)  [unwired: 1 in]
            n261 = Number To Decimal String(number=w423) -> (decimal integer string=w420:string)  [unwired: 1 in]
            n262 = Number To Decimal String(number=w424) -> (decimal integer string=w408:string)  [unwired: 1 in]
            n263 = call <vilib>:"Space Constant.vi"() -> ("String"=w421:string)
            n264 = Concatenate Strings(w407, "Data was taken on ", w418, w407, "Integration Time is ", w419, w421, "s", w407, "Monochromator gratng # ", w420, "; ", "blazed for ", w408, w421, "nm", w407, w407, w407, w406) -> (w422:string)
            n265 = Write to Text File(text=w422) -> ()  [unwired: 3 in, 3 out]
          }
        }
      }
    }
  }
  n266 = call "Configure.vi"("Dwell Time (s)"="Time between measurements\n at one point (s)/Dwell Time", "Channel T Input"="Trigger mode", "Channel B Input"="Channel B Input", "Channel A Input"="Channel A Input", "Integrating time, 10^-7 sec"="Integrating time \nin 10^-7 sec", "gate mode (CW:0)"="gate mode (CW:0)", "Scan End Mode"=FALSE, "Number of Periods"="Number of Measurements\n to take at one point/ Number of Periods", "Count Mode"="Count Mode", "GPIB Address"="GPIB address") -> ()
  "Mono port" <- w20
  "Time delay" <- w21
